vi "YAFTAF_SetExternalInterfaces.vi"(8 "ErrorIn":errorcluster, 10 "CmdData":variant, 11 "LocalIn":refnum<class>) -> (0 "ErrorOut":errorcluster, 2 "ReplyData":variant, 3 "LocalIn":refnum<class>, 4 "Exit":bool)   [LabVIEW 2021, in "YAFTAF.lvclass"]
uses:
  YAFTAF.lvclass
  Library_TAF_Support/ClusterArrayConversion/BundledArray.ctl
  Library_TAF_Support/ClusterArrayConversion/ClusterArrayConversion.lvlib
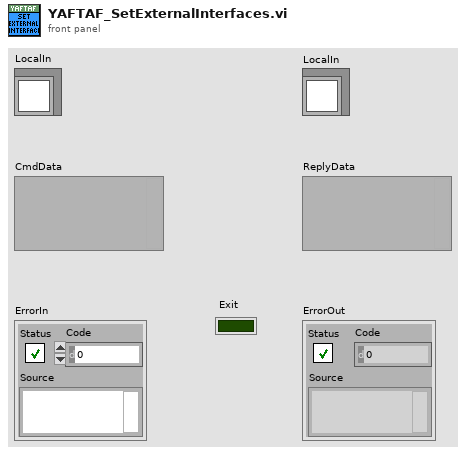
[diagram p1: front panel]
types:
  T1 = typedef "ClusterArrayConversion.lvlib/BundledArray.ctl" = cluster{"Label":string, "Object":refnum<class>, "Array":bool}
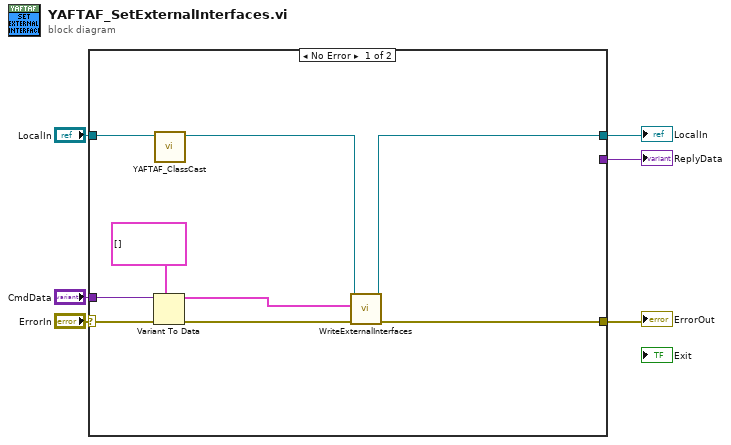
[diagram p0: block diagram]
diagram:
  n1 = case shown="No Error" "ErrorIn" {
    selector: "ErrorIn" -> [w15 w18]
    tunnel: [w14 w18] -> w5
    tunnel: [_ w17] -> w3
    tunnel: "CmdData" -> [w11 w17]
    tunnel: "LocalIn" -> [w12 w16]
    tunnel: [w8 w16] -> w1
    frame No Error {
      n2 = Variant To Data(error in=w15, type=T1[] [] ("ExternalInterfaces"), Variant=w11) -> (data=w7:T1[], error out=w13:errorcluster)
      n3 = call "YAFTAF_ClassCast.vi"("LocalIn"=w12) -> ("LocalOut"=w9:refnum<class "YAFTAF.lvclass">)  [unwired: 10 in]
      n4 = call-dynamic "WriteExternalInterfaces.vi"("ErrorIn"=w13, "ExternalInterfaces"=w7, "ObjectIn"=w9) -> ("ErrorOut"=w14:errorcluster, "ObjectOut"=w8:refnum<class "YAFTAF.lvclass">)  [unwired: 7 in]
    }
    frame Error {
    }
  }
  "ErrorOut" <- w5
  "LocalIn" <- w1
  "ReplyData" <- w3
